vi "Main_OnlyRFSG_SingleRecipe.vi"() -> ()   [LabVIEW 2014]
uses:
  15_DataManagement/Device_Resources.ctl
panel:
  in  "Device Resources":T1={"RFSG Resource in"="VST", "RFSA Resource in"="VST", "RFmx Resource in"="VST"}
  # "[ Single Receipe RFSG ]"
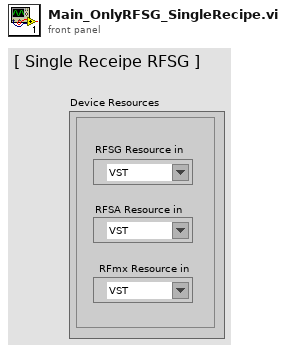
[diagram p1: front panel]
types:
  T1 = typedef "Device_Resources.ctl" = cluster{"RFSG Resource in":refnum<k15>, "RFSA Resource in":refnum<k15>, "RFmx Resource in":refnum<k15>}
  T2 = typedef "Message_Queues.ctl" = cluster{"RFSG_QTx":refnum<queue>, "RFSG_QRx":refnum<queue>, "RFSA_QTx":refnum<queue>, "RFSA_QRx":refnum<queue>, "SysLog":refnum<queue>, "RFSA_Data":refnum<queue>, "RFmx_QTx":refnum<queue>, "RFmx_QRx":refnum<queue>, "RFmx_Data":refnum<queue>}
  T3 = enum32{"Invalid", "Standard", "Closed", "Hidden", "Minimized", "Maximized"}
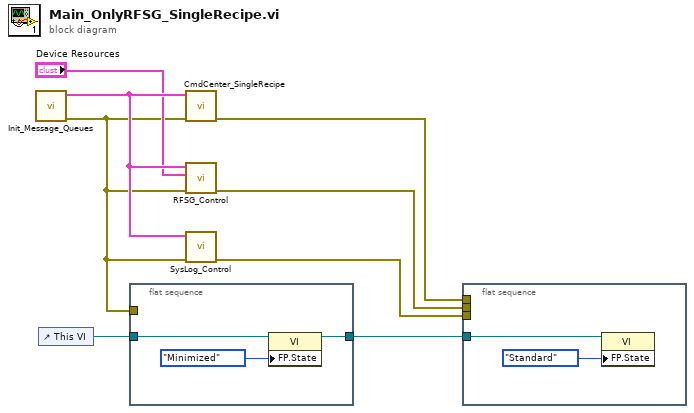
[diagram p0: block diagram]
diagram:
  n1 = call "Init_Message_Queues.vi"() -> ("error out"=w5:errorcluster, "Queue_Out"=w8:T2)  [unwired: 10 in]
  n2 = control-ref of="This VI"() -> (w6:refnum<vi>)
  n3 = flat-sequence {
    tunnel: w6 -> [w11]
    tunnel: w5 -> [_]
    tunnel: [w9] -> w4
    frame #0 {
      n4 = property class="VI"(reference=w11, "FP.State"=T3."Minimized" ("Front Panel Window:State")) -> (reference out=w9:refnum<vi>)  [unwired: 1 in, 1 out]
    }
  }
  n5 = call "CmdCenter_SingleRecipe.vi"("error in (no error)"=w5, "Message_Queues"=w8) -> ("error out"=w3:errorcluster)  [unwired: 9 in]
  n6 = call "RFSG_Control.vi"("error in (no error)"=w5, "Device Resources"="Device Resources", "Message_Queues"=w8) -> ("error out"=w2:errorcluster)  [unwired: 8 in]
  n7 = call "SysLog_Control.vi"("error in (no error)"=w5, "Message_Queues"=w8) -> ("error out"=w1:errorcluster)  [unwired: 9 in]
  n8 = flat-sequence {
    tunnel: w4 -> [w13]
    tunnel: w3 -> [_]
    tunnel: w2 -> [_]
    tunnel: w1 -> [_]
    frame #0 {
      n9 = property class="VI"(reference=w13, "FP.State"=T3."Standard" ("Front Panel Window:State")) -> ()  [unwired: 1 in, 2 out]
    }
  }
